vi "ChessEND.vi"(5 "ChessBoard in":T1, 9 "StoneColor":u16) -> (8 "ChessEND?":bool)   [LabVIEW 2009]
uses:
  Controls/Chess.ctl
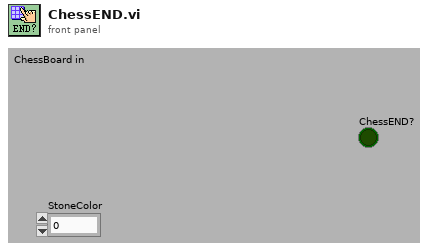
[diagram p1: front panel]
types:
  T1 = typedef "Chess.ctl" = u16[][]
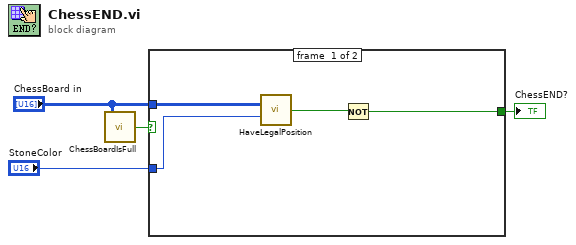
[diagram p0: block diagram]
diagram:
  n1 = call "ChessBoardIsFull.vi"("ChessBoard"="ChessBoard in") -> ("Full?"=w2:bool)  [unwired: 14 in]
  n2 = case shown="False" w2 {
    selector: w2 -> [_ w9]
    tunnel: "ChessBoard in" -> [w8 _]
    tunnel: [w5 w9] -> w1
    tunnel: "StoneColor" -> [w7 _]
    frame #0 {
      n3 = call "HaveLegalPosition.vi"("ChessBoard"=w8, "StoneColor"=w7) -> ("HaveLegalPlace?"=w6:bool)  [unwired: 13 in]
      n4 = Not(x=w6) -> (.not. x?=w5:bool)
    }
    frame #1 {
    }
  }
  "ChessEND?" <- w1
